vi "Step Flow.vi"(8 "error in (no error)":errorcluster, 11 "Step in":refnum<class "Step.lvclass">) -> (0 "error out":errorcluster, 3 "Step out":refnum<class "Step.lvclass">)   [LabVIEW 2015, in "Step.lvclass"]
uses:
  Step.lvclass
  Step Flow Control.ctl
  Step.lvclass/Step.ctl
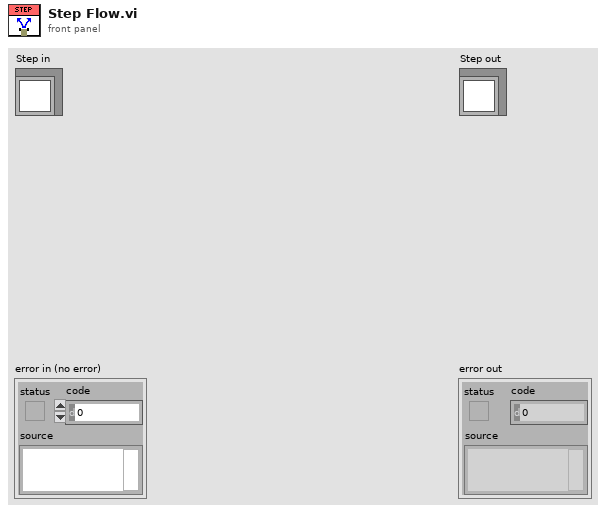
[diagram p1: front panel]
types:
  T1 = typedef "Step.lvclass/Step Flow Control.ctl" = enum16{"Next Step", "Jump"}
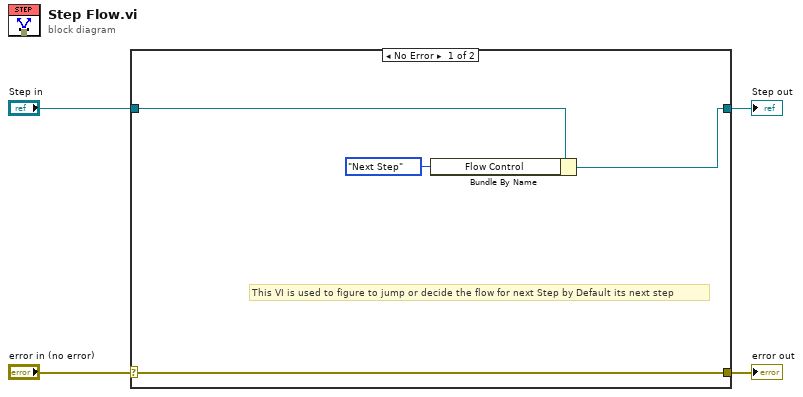
[diagram p0: block diagram]
diagram:
  n1 = case shown="No Error" "error in (no error)" {
    selector: "error in (no error)" -> [w8 w10]
    tunnel: [w8 w10] -> w3
    tunnel: [w6 w9] -> w1
    tunnel: "Step in" -> [w7 w9]
    frame No Error {
      # "This VI is used to figure to jump or decide the flow for next Step by Default its next step"
      n2 = Bundle By Name(cluster=w7, "Flow Control"=Step_Flow_Control."Next Step" ("Step State.Flow Control")) -> (w6:refnum<class "Step.lvclass">)
    }
    frame Error {
    }
  }
  "error out" <- w3
  "Step out" <- w1
